vi "rank.vi"(1 "玩家名称":string, 2 "得分":i64) -> ()   [LabVIEW 2011]
uses:
  <vilib>/Utility/file.llb/Read From Spreadsheet File (string).vi
  <vilib>/Utility/file.llb/Write To Spreadsheet File (string).vi
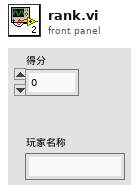
[diagram p1: front panel]
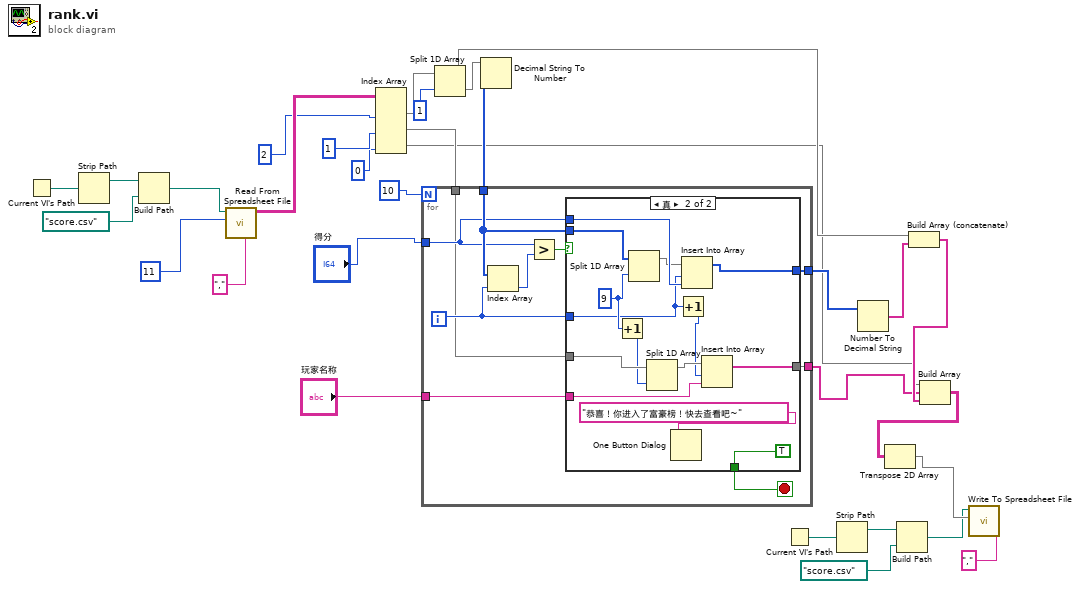
[diagram p0: block diagram]
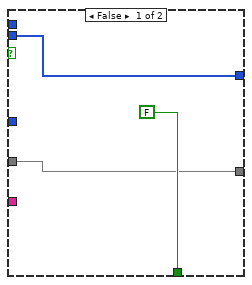
[diagram p2: hidden frame]
diagram:
  n1 = Current VI's Path() -> (path=w8:path)
  n2 = Strip Path(path=w8) -> (stripped path=w7:path)  [unwired: 1 out]
  n3 = Build Path(base path=w7, name or relative path=path "score.csv") -> (appended path=w5:path)
  n4 = call-poly <vilib>:"Read From Spreadsheet File.vi"("delimiter (\\t)"=",", "number of rows (all:-1)"=11, "file path (dialog if empty)"=w5) -> ("all rows"=w29:string[][])  [unwired: 4 in, 4 out]
  n5 = Index Array(array=w29, index (col) #1=2, index (col) #2=1, index (col) #3=0) -> (element #1=w19:string[], element #2=w24:string[], element #3=w11:string[])  [unwired: 3 in]
  n6 = Split 1D Array(array=w19, index=1) -> (first subarray=w16:string[], second subarray=w17:string[])
  n7 = Decimal String To Number(string=w17) -> (number=w26:i32[])  [unwired: 2 in, 1 out]
  n8 = for {
    N: 10 -> [_]
    tunnel: w26 -> [w39]
    tunnel: "得分" -> [w38]
    tunnel: [w37] -> w23
    tunnel: w24 -> [w34]
    tunnel: "玩家名称" -> [w33]
    tunnel: [w32] -> w12
    i -> [w35]
    stop <- w36 stop-if-true
    n9 = Index Array ("索引数组")(array=w39, index=w35) -> (element=w41:i32)
    n10 = Greater?(x=w38, y=w41) -> (0:w40:bool)
    n11 = case shown="真" w40 {
      tunnel: w39 -> [w43 w57]
      tunnel: w35 -> [_ w46]
      tunnel: w38 -> [_ w58]
      tunnel: [w43 w55] -> w37
      tunnel: [FALSE TRUE] -> w36
      tunnel: w34 -> [w42 w53]
      tunnel: w33 -> [_ w51]
      tunnel: [w42 w50] -> w32
      frame False {
      }
      frame True {
        w48 = 9
        n12 = Increment(x=w48) -> (x+1=w47:i32)
        n13 = Split 1D Array(array=w57, index=w48) -> (first subarray=w56:i32[])  [unwired: 1 out]
        n14 = Split 1D Array(array=w53, index=w47) -> (first subarray=w52:string[])  [unwired: 1 out]
        n15 = One Button Dialog(message="恭喜！你进入了富豪榜！快去查看吧~") -> ()  [unwired: 1 in, 1 out]
        n16 = Increment(x=w46) -> (x+1=w45:i32)
        n17 = Insert Into Array(array=w56, index=w46, new element=w58) -> (w55:i32[])
        n18 = Insert Into Array(array=w52, index=w45, new element=w51) -> (w50:string[])
      }
    }
  }
  n19 = Current VI's Path() -> (path=w4:path)
  n20 = Strip Path(path=w4) -> (stripped path=w3:path)  [unwired: 1 out]
  n21 = Number To Decimal String(number=w23) -> (decimal integer string=w14:string[])  [unwired: 1 in]
  n22 = Build Path(base path=w3, name or relative path=path "score.csv") -> (appended path=w1:path)
  n23 = Build Array (concatenate)(w16, w14) -> (w13:string[])
  n24 = Build Array(w11, w12, w13) -> (w22:string[][])
  n25 = Transpose 2D Array(2D array=w22) -> (transposed array=w21:string[][])
  n26 = call-poly <vilib>:"Write To Spreadsheet File.vi"("delimiter (\\t)"=",", "2D data"=w21, "file path (dialog if empty)"=w1) -> ()  [unwired: 5 in, 1 out]
